vi "fileLoadFloatVector.vi"(11 "File Path":path) -> (0 "error out":errorcluster, 3 "Float Vector":dbl[](array[numeric]))   [LabVIEW 2010, in "kevLib2011.lvlib"]
uses:
  kevLib2011.lvlib
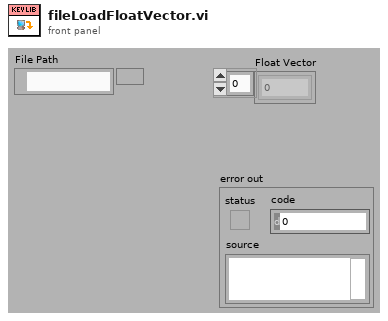
[diagram p1: front panel]
types:
  T1 = enum16{"open", "replace", "create", "open or create", "replace or create", "replace or create with confirmation"}
  T2 = enum16{"deny read/write", "deny write-only", "deny none"}
  T3 = enum16{"big-endian, network order", "native, host order", "little-endian"}
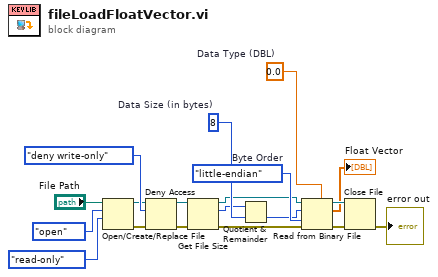
[diagram p0: block diagram]
diagram:
  w12 = T3."little-endian"  # Byte Order
  w10 = i64 8  # Data Size (in bytes)
  w9 = 0.0  # Data Type (DBL)
  n1 = Open/Create/Replace File(file path (use dialog)="File Path", operation (0:open)=T1."open", access (0:read/write)=enum16{"read/write", "read-only", "write-only"}."read-only") -> (refnum out=w14:refnum<file>, error out=w13:errorcluster)  [unwired: 1 in, 3 out]
  n2 = Deny Access(4:w13, 6:T2."deny write-only" ("deny mode (0:deny read/write)"), 7:w14) -> (0:w15:errorcluster, 3:w16:refnum<file>)
  n3 = Get File Size(file=w16, error in=w15) -> (refnum out=w3:refnum<file>, size (in bytes)=w6:i64, 0:w7:errorcluster)
  n4 = Quotient & Remainder(x=w6, y=w10) -> (floor(x/y)=w11:i64)  [unwired: 1 out]
  n5 = Read from Binary File(5:w9, 8:w7, 9:w12, 10:w11, 11:w3) -> (0:w5:errorcluster, 2:→"Float Vector":dbl[], 3:w4:refnum<file>)  [unwired: 2 out]
  n6 = Close File(refnum=w4, error in=w5) -> (error out=→"error out":errorcluster)  [unwired: 1 out]
